vi "Broker.vi"() -> ()   [LabVIEW 2022 SP3]
uses:
  <vilib>/G Open Source Project for LabVIEW/MQTT Broker/Server class/Server.lvclass/Server.ctl
  <vilib>/LabVIEW Open Source Project/MQTT TCP Connection/MQTT_TCP/Connection/TCPConnection.lvclass
  C:/Program Files/National Instruments/LabVIEW 2022/vi.lib/LabVIEW Open Source Project/Connection/Connection/Connection.lvclass
  <vilib>/G Open Source Project for LabVIEW/MQTT Broker/Server class/Server.lvclass
  C:/Program Files/National Instruments/LabVIEW 2022/vi.lib/LabVIEW Open Source Project/MQTT Connection/MQTT_Base/Base Class/MQTT_Base.lvclass
  <vilib>/LabVIEW Open Source Project/MQTT Connection/MQTT_Base/Base Class/MQTT_Base.lvclass
panel:
  out "NbConnections":u32
  out "error server":errorcluster
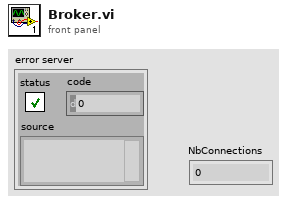
[diagram p1: front panel]
types:
  T1 = typedef "MQTT Server.lvlib/Server.lvclass/Public Events -- cluster.ctl" = cluster{"NbConnections":refnum<user-event>, "Client Event":refnum<user-event>}
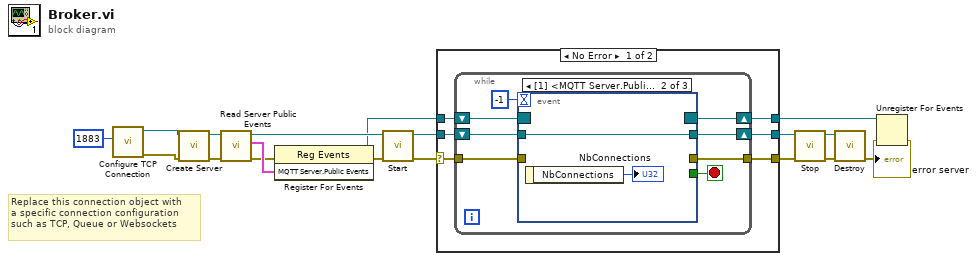
[diagram p0: block diagram]
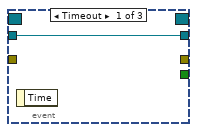
[diagram p2: hidden frame]
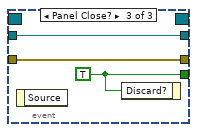
[diagram p3: hidden frame]
diagram:
  # "Replace this connection object with\na specific connection configuration\nsuch as TCP, Queue or Websockets"
  n1 = call <vilib>:"Configure TCP Connection.vi"("remote port (80)"=u16 1883) -> ("error out"=w1:errorcluster, "TCPConnection"=w2:refnum<class "TCPConnection.lvclass">)  [unwired: 9 in]
  n2 = call <vilib>:"Create Server.vi"("error in (no error)"=w1, "Connection Configuration"=w2) -> ("error out"=w5:errorcluster, "Server"=w4:refnum<class "Server.lvclass">)  [unwired: 8 in]
  n3 = call <vilib>:"Read Server Public Events.vi"("error in (no error)"=w5, "Server in"=w4) -> ("error out"=w6:errorcluster, "MQTT Server.Public Events"=w7:T1, "Server out"=w10:refnum<class "Server.lvclass">)  [unwired: 7 in]
  n4 = register-events(error in=w6, w7) -> (reference out=w8:refnum<event-registration>, error out=w12:errorcluster)  [unwired: 1 in]
  n5 = call <vilib>:"Start.vi"("error in (no error)"=w12, "MQTT_Base in"=w10) -> ("error out"=w13:errorcluster, "MQTT_Base out"=w11:refnum<class "Server.lvclass">)  [unwired: 7 in, 1 out]
  n6 = case shown="No Error" w13 {
    selector: w13 -> [w19 w39]
    tunnel: w11 -> [w24 w41]
    tunnel: [w23 w41] -> w16
    tunnel: w8 -> [w22 w40]
    tunnel: [w21 w40] -> w9
    tunnel: [w20 w39] -> w18
    frame No Error {
      n7 = while {
        shift-right: [w29] -> w23
        shift-left: w24 -> [w31]
        tunnel: [w26] -> w20
        tunnel: w19 -> [w25]
        shift-right: [w27] -> w21
        shift-left: w22 -> [w28]
        stop <- w30 stop-if-true
        n8 = event shown="[1] <MQTT Server.Public Events.NbConnections>: User Event" {
          selector: w28 -> [_ _ _]
          dyn-events: [_ _ _] -> w27
          timeout: -1 -> [_ _ _]
          tunnel: w31 -> [w33 w35 w38]
          tunnel: [_ _ w36] -> w30
          tunnel: [w33 w35 w38] -> w29
          tunnel: [_ _ w37] -> w26
          tunnel: w25 -> [_ _ w37]
          event Timeout {
            n9 = event-data() -> ()  [unwired: 1 in, 1 out]
          }
          event User Event {
            n10 = event-data() -> ("NbConnections"=→"NbConnections":u32)  [unwired: 1 in]
          }
          event Panel Close? {
            w36 = TRUE ("Discard?")
            n11 = event-data() -> ()  [unwired: 1 in, 1 out]
            n12 = event-data("Discard?"=w36) -> ()  [unwired: 1 in, 1 out]
          }
        }
      }
    }
    frame Error {
    }
  }
  n13 = call <vilib>:"Stop.vi"("error in (no error)"=w18, "MQTT_Base in"=w16) -> ("error out"=w17:errorcluster, "MQTT_Base out"=w15:refnum<class "Server.lvclass">)  [unwired: 7 in, 1 out]
  n14 = call <vilib>:"Destroy.vi"("error in (no error)"=w17, "MQTT_Base in"=w15) -> ("error out"=→"error server":errorcluster)  [unwired: 8 in, 1 out]
  n15 = Unregister For Events(event registration refnum=w9) -> ()  [unwired: 1 in, 1 out]
